vi "Configure.vi"(8 "error in (no error)":errorcluster, 11 "ImageHandler in":refnum<class "ImageHandler.lvclass">) -> (0 "error out":errorcluster, 3 "ImageHandler out":refnum<class "ImageHandler.lvclass">)   [LabVIEW 2022 SP3, in "ImageHandler.lvlib" / "ImageHandler.lvclass"]
uses:
  ImageHandler.lvclass
  ImageHandler.lvclass/ImageHandler.ctl
  BonTechDetector/BonTechDetector.lvlib
panel:
  out "nHeight out":u16
  out "nWidth out":u16
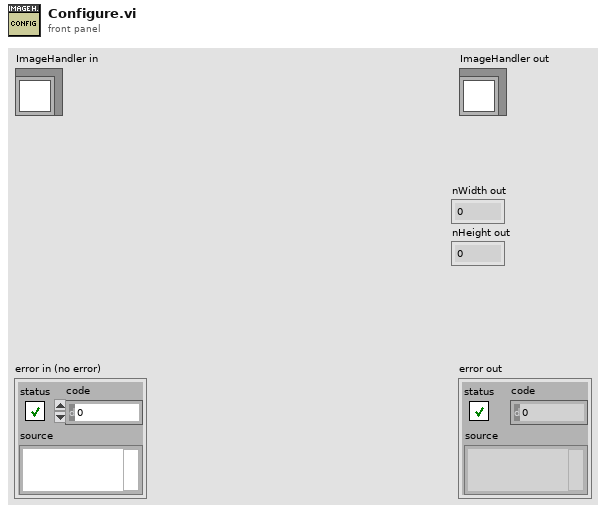
[diagram p1: front panel]
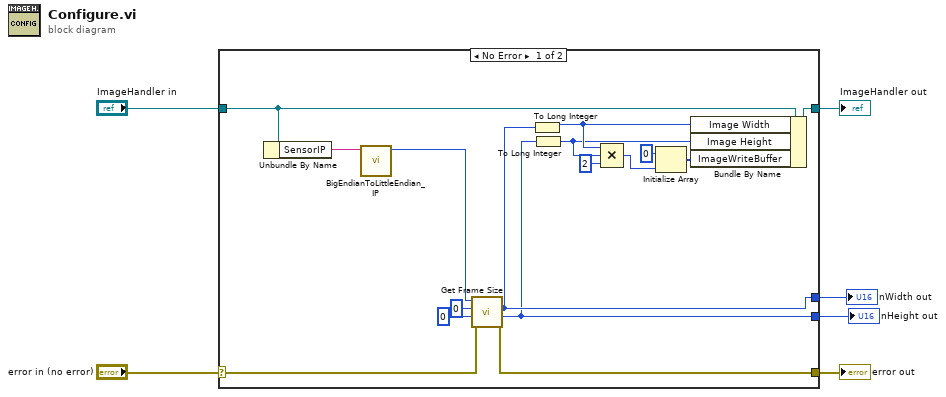
[diagram p0: block diagram]
diagram:
  n1 = case shown="No Error" "error in (no error)" {
    selector: "error in (no error)" -> [w20 w24]
    tunnel: [w19 w24] -> w5
    tunnel: [w15 w23] -> w3
    tunnel: "ImageHandler in" -> [w22 w23]
    tunnel: [w13 _] -> w2
    tunnel: [w14 _] -> w1
    frame No Error {
      n2 = Unbundle By Name(w22) -> ("SensorIP"=w21:string)
      n3 = call "BigEndianToLittleEndian_IP.vi"("IP String"=w21) -> ("IP Network Order"=w16:u32)  [unwired: 10 in]
      n4 = call "Get Frame Size.vi"("error in (no error)"=w20, "nHeight"=u16 0, "nWidth"=u16 0, "nSensorIP"=w16) -> ("error out"=w19:errorcluster, "nHeight out"=w13:u16, "nWidth out"=w14:u16)  [unwired: 4 in, 1 out]
      n5 = To Long Integer(number=w14) -> (32bit integer=w12:i32)
      n6 = To Long Integer(number=w13) -> (32bit integer=w11:i32)
      n7 = Compound Arithmetic op=MULTIPLY(w12, w11, 2 ("value")) -> (w8:i32)
      n8 = Initialize Array(u16 0, w8) -> (w9:u16[])
      n9 = Bundle By Name(cluster=w22, "Image Width"=w12, "Image Height"=w11, "ImageWriteBuffer"=w9) -> (w15:refnum<class "ImageHandler.lvclass">)
    }
    frame Error {
    }
  }
  "error out" <- w5
  "ImageHandler out" <- w3
  "nWidth out" <- w1
  "nHeight out" <- w2
